vi "Sort Objects.vi"(0 "Object List in":i32[][](array[numeric]), 5 "error in (no error)":errorcluster) -> (14 "Object List out":i32[][](array[numeric]), 19 "error out":errorcluster)   [LabVIEW 2016]
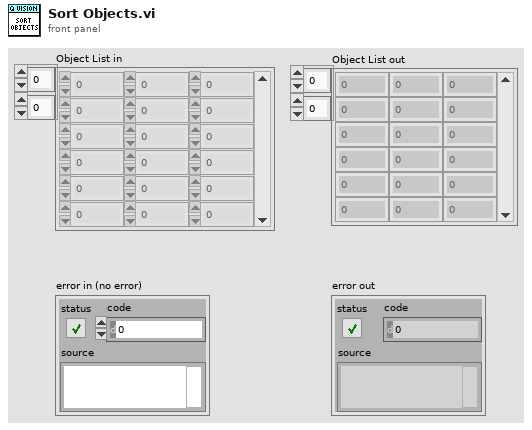
[diagram p1: front panel]
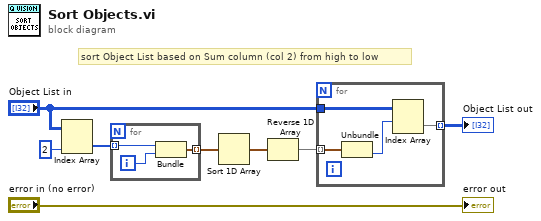
[diagram p0: block diagram]
diagram:
  # "sort Object List based on Sum column (col 2) from high to low"
  n1 = Index Array(array="Object List in", index (col)=2 ("disabled index (col)")) -> (element=w6:i32[])  [unwired: 1 in]
  n2 = for {
    tunnel: w6 -> [w11] mode=indexing
    tunnel: [w9] -> w5 mode=indexing
    i -> [w10]
    n3 = Bundle("Numeric"=w11, w10) -> (w9:cluster{"Numeric":i32, i32})  [unwired: 1 in]
  }
  n4 = Sort 1D Array(array=w5) -> (sorted array=w4:cluster{"Numeric":i32, i32}[])
  n5 = Reverse 1D Array(array=w4) -> (reversed array=w3:cluster{"Numeric":i32, i32}[])
  n6 = for {
    tunnel: w3 -> [w15] mode=indexing
    tunnel: "Object List in" -> [w14]
    tunnel: [w12] -> w1 mode=indexing
    n7 = Unbundle(w15) -> (w13:i32)  [unwired: 1 out]
    n8 = Index Array(array=w14, index (row)=w13) -> (element=w12:i32[])  [unwired: 1 in]
  }
  "Object List out" <- w1
  "error out" <- "error in (no error)"
